vi "FrequencyXlation.vi"() -> ()   [LabVIEW 2009]
uses:
  <vilib>/imath/engines/lvmath2/RunTimeEngine/ErrorHandling/NIMS_Finalize Error.vi
  <vilib>/imath/engines/lvmath2/RunTimeEngine/Parser/MC_Version.vi
  <vilib>/imath/engines/lvmath2/RunTimeEngine/NodeEndStatement/NIMS_NodeEndStatement_Output.vi
  <instcachedir>/0/NIMS_NodeEndStatement_Output_53EC0D466D134D7ABD903AC30B43404B.lvgen/NIMS_NodeEndStatement_Output_53EC0D466D134D7ABD903AC30B43404B_001.vi
  <vilib>/imath/engines/lvmath2/RunTimeEngine/RangeToken/NIMS_Range.vi
  <instcachedir>/0/NIMS_Range_08574DECC23E450FAF0AC0BC39E6BEA7.lvgen/NIMS_Range_08574DECC23E450FAF0AC0BC39E6BEA7_001.vi
  <vilib>/imath/engines/lvmath/Functions/Error Handling/MergeErrorsWrapper.vi
  <vilib>/imathl/engines/lvmath/Functions/Error Handling/Create Error.vi
  <vilib>/imath/engines/lvmath/Functions/Error Handling/MC_Error Cluster From Error Code.vi
  <vilib>/imath/engines/lvmath2/RunTimeEngine/BuiltInFunctions/rand/NIMS_rand(1,I32).vi
  <vilib>/imath/engines/lvmath2/RunTimeEngine/ArithmeticOperatorToken/NIMS_ArithmeticOperator_plus.vi
  <instcachedir>/0/NIMS_ArithmeticOperator_plus_48B9519178ED42D7840F01273E784BFE.lvgen/NIMS_ArithmeticOperator_plus_48B9519178ED42D7840F01273E784BFE_000.vi
  <vilib>/imath/engines/lvmath2/RunTimeEngine/BuiltInFunctions/abs/NIMS_abs(signed).vi
  <instcachedir>/0/NIMS_abs(signed)_C4FCB8E6058B49B797C7C8D53CA5F6EC.lvgen/NIMS_abs(signed)_C4FCB8E6058B49B797C7C8D53CA5F6EC_000.vi
  <vilib>/imath/engines/lvmath2/RunTimeEngine/BuiltInFunctions/fft/NIMS_fft(GV).vi
  <instcachedir>/0/NIMS_fft(GV)_4C6467FC22F84E4BA42517A07EF978B0.lvgen/NIMS_fft(GV)_4C6467FC22F84E4BA42517A07EF978B0_001.vi
  <vilib>/imath/engines/lvmath2/RunTimeEngine/BuiltInFunctions/zeros/NIMS_V=zeros(I32,I32).vi
  <vilib>/imath/engines/lvmath2/RunTimeEngine/RangeToken/NIMS_Range_R2 - Float.vi
  <instcachedir>/0/NIMS_Range_R2 - Float_93A1434467634702BCAD427B3499A8B4.lvgen/NIMS_Range_R2 - Float_93A1434467634702BCAD427B3499A8B4_000.vi
  <vilib>/imath/engines/lvmath2/RunTimeEngine/ReplaceToken/NIMS_Replace - V(S)=S.vi
  <instcachedir>/0/NIMS_Replace - V(S)=S_1F711D65782C407D901BB57589CB2660.lvgen/NIMS_Replace - V(S)=S_1F711D65782C407D901BB57589CB2660_001.vi
  <vilib>/imath/engines/lvmath2/RunTimeEngine/ReplaceToken/NIMS_Replace - Size Check _(_)=S.vi
  <instcachedir>/0/NIMS_Replace - Size Check _(_)=S_C93E24300E2D4FA1B1057E3B3E42F8F7.lvgen/NIMS_Replace - Size Check _(_)=S_C93E24300E2D4FA1B1057E3B3E42F8F7_001.vi
  <vilib>/imath/engines/lvmath2/RunTimeEngine/VariableToken/Read/NIMS_Get Elements - RV(_) - Check(_).vi
  <instcachedir>/0/NIMS_Get Elements - RV(_) - Check(_)_FD08F12CA9A340B3A4DC1D5FF02404A0.lvgen/NIMS_Get Elements - RV(_) - Check(_)_FD08F12CA9A340B3A4DC1D5FF02404A0_001.vi
  <vilib>/imath/engines/lvmath2/RunTimeEngine/ArithmeticOperatorToken/NIMS_ArithmeticOperator_power(S).vi
  <instcachedir>/0/NIMS_ArithmeticOperator_power(S)_4AA2794EBDEE41D3AEDF40937D3906E7.lvgen/NIMS_ArithmeticOperator_power(S)_4AA2794EBDEE41D3AEDF40937D3906E7_002.vi
  <vilib>/imath/engines/lvmath2/RunTimeEngine/ReplaceToken/NIMS_Replace - Check(_) Linear.vi
  <instcachedir>/0/NIMS_Replace - Check(_) Linear_E275C9AF2D6949DA8BBA624A5DF43407.lvgen/NIMS_Replace - Check(_) Linear_E275C9AF2D6949DA8BBA624A5DF43407_003.vi
  <vilib>/imath/engines/lvmath2/RunTimeEngine/CommandStatement/MC_CommandStatement_break.vi
  <instcachedir>/0/NIMS_fft(GV)_4C6467FC22F84E4BA42517A07EF978B0.lvgen/NIMS_fft(GV)_4C6467FC22F84E4BA42517A07EF978B0_000.vi
  <instcachedir>/0/NIMS_Replace - V(S)=S_1F711D65782C407D901BB57589CB2660.lvgen/NIMS_Replace - V(S)=S_1F711D65782C407D901BB57589CB2660_000.vi
  <instcachedir>/0/NIMS_Replace - Size Check _(_)=S_C93E24300E2D4FA1B1057E3B3E42F8F7.lvgen/NIMS_Replace - Size Check _(_)=S_C93E24300E2D4FA1B1057E3B3E42F8F7_002.vi
  <instcachedir>/0/NIMS_Replace - Check(_) Linear_E275C9AF2D6949DA8BBA624A5DF43407.lvgen/NIMS_Replace - Check(_) Linear_E275C9AF2D6949DA8BBA624A5DF43407_004.vi
panel:
  out "Xlated by fs/4":dbl[](graph)
  out "Xlated by fs/2":dbl[](graph)
  out "Original signal":dbl[](graph)
  in  "M3":dbl=12.0
  in  "M2":dbl=11.0
  in  "M1":dbl=10.0
  in  "N":dbl=64.0
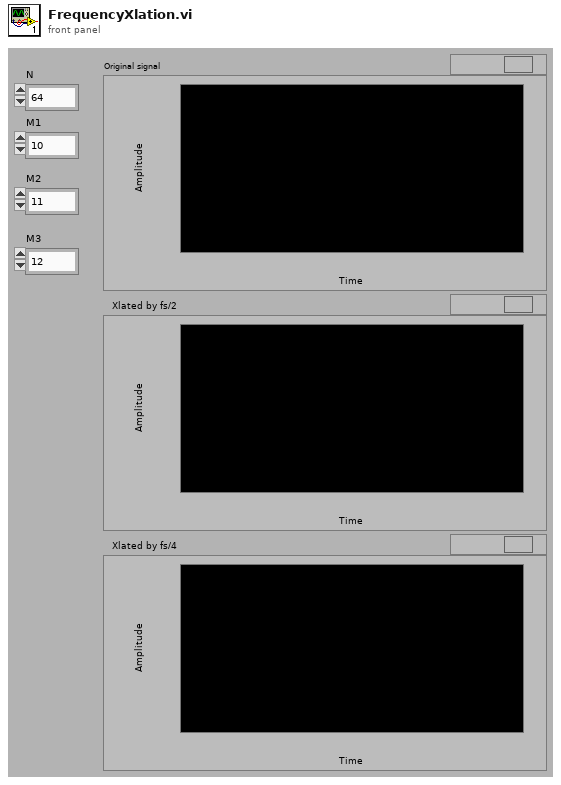
[diagram p1: front panel]
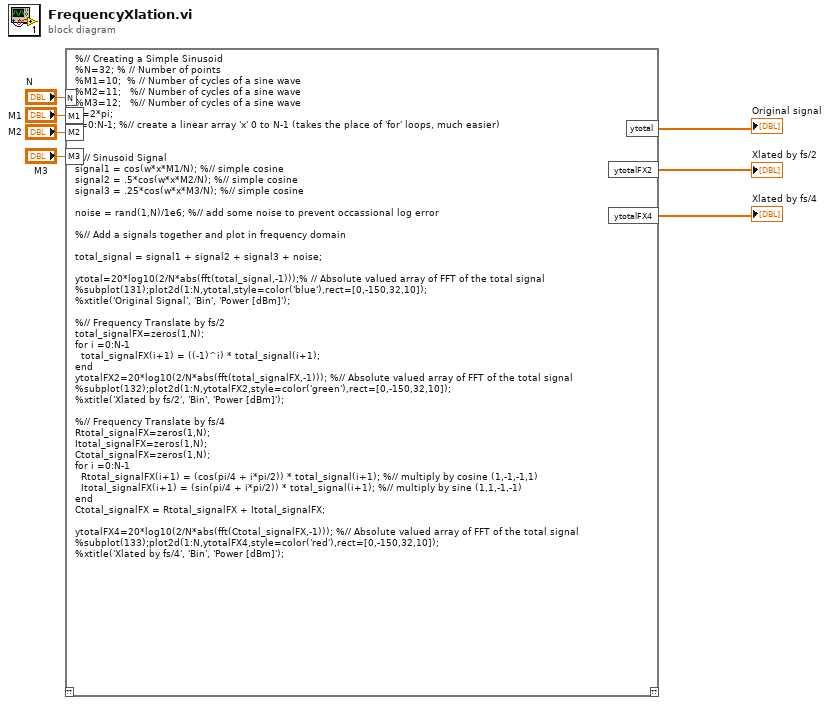
[diagram p0: block diagram]
diagram:
  n1 = mathscript code="%// Creating a Simple Sinusoid\n%N=32; % // Number of points\n%M1=10;  % // Number of cycles of a sine wave\n%M2=11;   %// Number of cycles of a sine wave\n%M3=12;   %// Number of cycles of a sine wave\nw=2*pi; \nx=0:N-1; %// create a linear array 'x' 0 to N-1 (takes the place of 'for' loops, much easier)\n\n\n%// Sinusoid Signal\nsignal1 = cos(w*x*M1/N); %// simple cosine\nsignal2 = .5*cos(w*x*M2/N); %// simple cosine\nsignal3 = .25*cos(w*x*M3/N); %// simple cosine\n\nnoise = rand(1,N)/1e6; %// add some noise to prevent occassional log error\n\n%// Add a signals together and plot in frequency domain\n\ntotal_signal = signal1 + signal2 + signal3 + noise;\n\nytotal=20*log10(2/N*abs(fft(total_signal,-1)));% // Absolute valued array of FFT of the total signal \n%subplot(131);plot2d(1:N,ytotal,style=color('blue'),rect=[0,-150,32,10]); \n%xtitle('Original Signal', 'Bin', 'Power [dBm]');\n\n%// Frequency Translate by fs/2\ntotal_signalFX=zeros(1,N);\nfor i =0:N-1\n  total_signalFX(i+1) = ((-1)^i) * total_signal(i+1);\nend\nytotalFX2=20*log10(2/N*abs(fft(total_signalFX,-1))); %// Absolute valued array of FFT of the total signal \n%subplot(132);plot2d(1:N,ytotalFX2,style=color('green'),rect=[0,-150,32,10]); \n%xtitle('Xlated by fs/2', 'Bin', 'Power [dBm]');\n\n%// Frequency Translate by fs/4\nRtotal_signalFX=zeros(1,N);\nItotal_signalFX=zeros(1,N);\nCtotal_signalFX=zeros(1,N);\nfor i =0:N-1\n  Rtotal_signalFX(i+1) = (cos(pi/4 + i*pi/2)) * total_signal(i+1); %// multiply by cosine (1,-1,-1,1)\n  Itotal_signalFX(i+1) = (sin(pi/4 + i*pi/2)) * total_signal(i+1); %// multiply by sine (1,1,-1,-1)\nend\nCtotal_signalFX = Rtotal_signalFX + Itotal_signalFX;\n\nytotalFX4=20*log10(2/N*abs(fft(Ctotal_signalFX,-1))); %// Absolute valued array of FFT of the total signal \n%subplot(133);plot2d(1:N,ytotalFX4,style=color('red'),rect=[0,-150,32,10]); \n%xtitle('Xlated by fs/4', 'Bin', 'Power [dBm]');"("N"="N", "M1"="M1", "M2"="M2", "M3"="M3") -> ("ytotal"=→"Original signal":dbl[], "ytotalFX2"=→"Xlated by fs/2":dbl[], "ytotalFX4"=→"Xlated by fs/4":dbl[])  [unwired: 1 in, 1 out]
